vi "LSX Set Language.vi"(8 "error in (no error)":errorcluster, 10 "pcPLN":string, 11 "lLSID":i32) -> (0 "error out":errorcluster, 2 "pcPLN out":string, 3 "function return":i32)   [LabVIEW 2018, in "Tango.lvlib"]
doc: "TANGOAPI int TANGOCALL LSX_SetLanguage (int lLSID, char *pcPLN);"
uses:
  Tango.lvlib
  SubVIs/Tango_DLL.dll
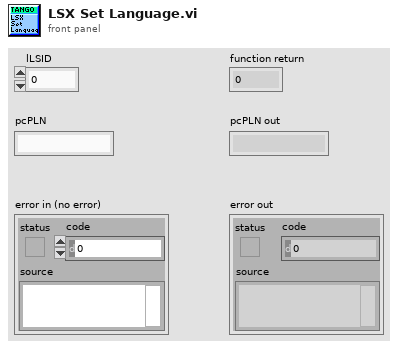
[diagram p1: front panel]
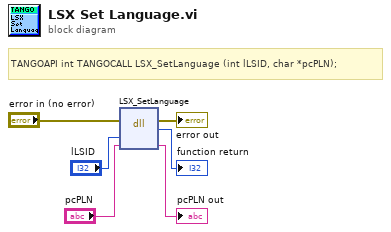
[diagram p0: block diagram]
diagram:
  # "TANGOAPI int TANGOCALL LSX_SetLanguage (int lLSID, char *pcPLN);"
  n1 = dll-call lib="C:/Users/Familie/Documents/LabviewIX81/lib/TANGO Stage/SubVIs/Tango_DLL.*" fn="LSX_SetLanguage"(error in="error in (no error)", "lLSID"="lLSID", "pcPLN"="pcPLN") -> (error out=→"error out":errorcluster, →"function return":i32, "pcPLN"=→"pcPLN out":string)  [unwired: 3 in, 1 out]
